vi "ConvertAFolderOfITXfiles.vi"() -> ()   [LabVIEW 2016]
panel:
  out "files converted":i32
  in  "Input ITX Folder":path=path "B:/SketchSET/SA03008H.20180718/21-BG+SG_Sweep+OVERNIGHT"
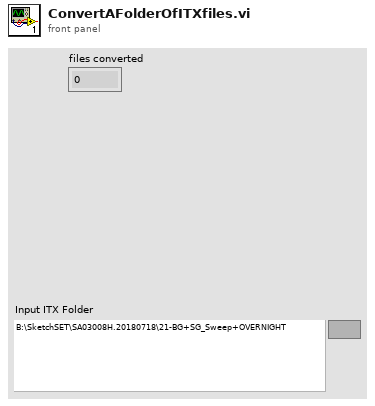
[diagram p1: front panel]
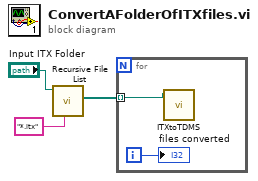
[diagram p0: block diagram]
diagram:
  n1 = call <vilib>:"Recursive File List.vi"("pattern"="*.itx", "Folder Path"="Input ITX Folder") -> ("All Files in Dir"=w1:path[])  [unwired: 5 in, 4 out]
  n2 = for {
    tunnel: w1 -> [w5] mode=indexing
    i -> [w4]
    n3 = call "ITXtoTDMS.vi"("Currrent ITX file 2"=w5) -> ()  [unwired: 11 in]
    "files converted" <- w4
  }
